vi "Outputs.vi"(8 "error in (no error)":errorcluster, 11 "State in":T1={"State"=enum."Idle", "Start Time"=timestamp(0 s since 1904-01-01), "Configuration"={"Cycle Period"=0.0, "Setpoint Entry"=0.0, "Output Device"=enum."Huber Ministat 230", "Huber Ministat 230 Settings"={"VISA resource name"="", "Simulated?"=FALSE}, "Lauda Settings"={"VISA resource name"="", "Simulated?"=FALSE, "Pump Power"=2}, "Julabo FP-50 Settings"={"VISA resource name"="", "Simulated?"=FALSE, "Pump Power"=2}, "Internal Control?"=FALSE, "Huber Unistat 410 Settings"={"VISA resource name"="", "Simulated?"=FALSE}}, "Current Time"=timestamp(0 s since 1904-01-01), "First Iteration"=FALSE, "Data"={"TCU Speed"=0.0, "Temperature"=0.0}, "Process Name"="", "TCU On?"=FALSE, "Output Error"=FALSE, "Start Log"=FALSE, "Power Level Changed"=FALSE} {"Configuration"."Julabo FP-50 Settings"."Pump Power" min=0 max=8 step=1; "Configuration"."Lauda Settings"."Pump Power" min=0 max=8 step=1}) -> (0 "error out":errorcluster, 3 "State out":T1={"State"=enum."Idle", "Start Time"=timestamp(0 s since 1904-01-01), "Configuration"={"Cycle Period"=0.0, "Setpoint Entry"=0.0, "Output Device"=enum."Huber Ministat 230", "Huber Ministat 230 Settings"={"VISA resource name"="", "Simulated?"=FALSE}, "Lauda Settings"={"VISA resource name"="", "Simulated?"=FALSE, "Pump Power"=2}, "Julabo FP-50 Settings"={"VISA resource name"="", "Simulated?"=FALSE, "Pump Power"=2}, "Internal Control?"=FALSE, "Huber Unistat 410 Settings"={"VISA resource name"="", "Simulated?"=FALSE}}, "Current Time"=timestamp(0 s since 1904-01-01), "First Iteration"=FALSE, "Data"={"TCU Speed"=0.0, "Temperature"=0.0}, "Process Name"="", "TCU On?"=FALSE, "Output Error"=FALSE, "Start Log"=FALSE, "Power Level Changed"=FALSE} {"Configuration"."Julabo FP-50 Settings"."Pump Power" min=0 max=8 step=1; "Configuration"."Lauda Settings"."Pump Power" min=0 max=8 step=1})   [LabVIEW 2018, in "TCU Module.lvlib" / "TCU Module Engine.lvlib"]
uses:
  TCU Module Engine.lvlib
  TCU State Cluster.ctl
  State Enum.ctl
  TCU Module Settings Cluster.ctl
  Output Devices.ctl
  Huber TCU/Huber Settings.ctl
  Lauda Integral XT-150 TCU/Lauda Settings.ctl
  Julabo Type 1 TCU/Julabo Type 1 TCU Folder/Julabo FP-50 Settings.ctl
  Huber Unistat 410 TCU/Huber Unistat 410 Settings.ctl
  Tag VIs/Tag FGV Operation Enum.ctl
  Shared Variables/Dynamic Shared Variables.lvlib
  Huber TCU/Huber Ministat 230 TCU.lvlib
  Lauda Integral XT-150 TCU/Lauda TCU.lvlib
  Julabo Type 1 TCU/Julabo Type 1 TCU Folder/Julabo Type FP-50 TCU.lvlib
  Huber Unistat 410 TCU/Huber Unistat 410 TCU.lvlib
  TCU Module.lvlib
panel:
  # "Output Instruments"
  # "Output Instruments"
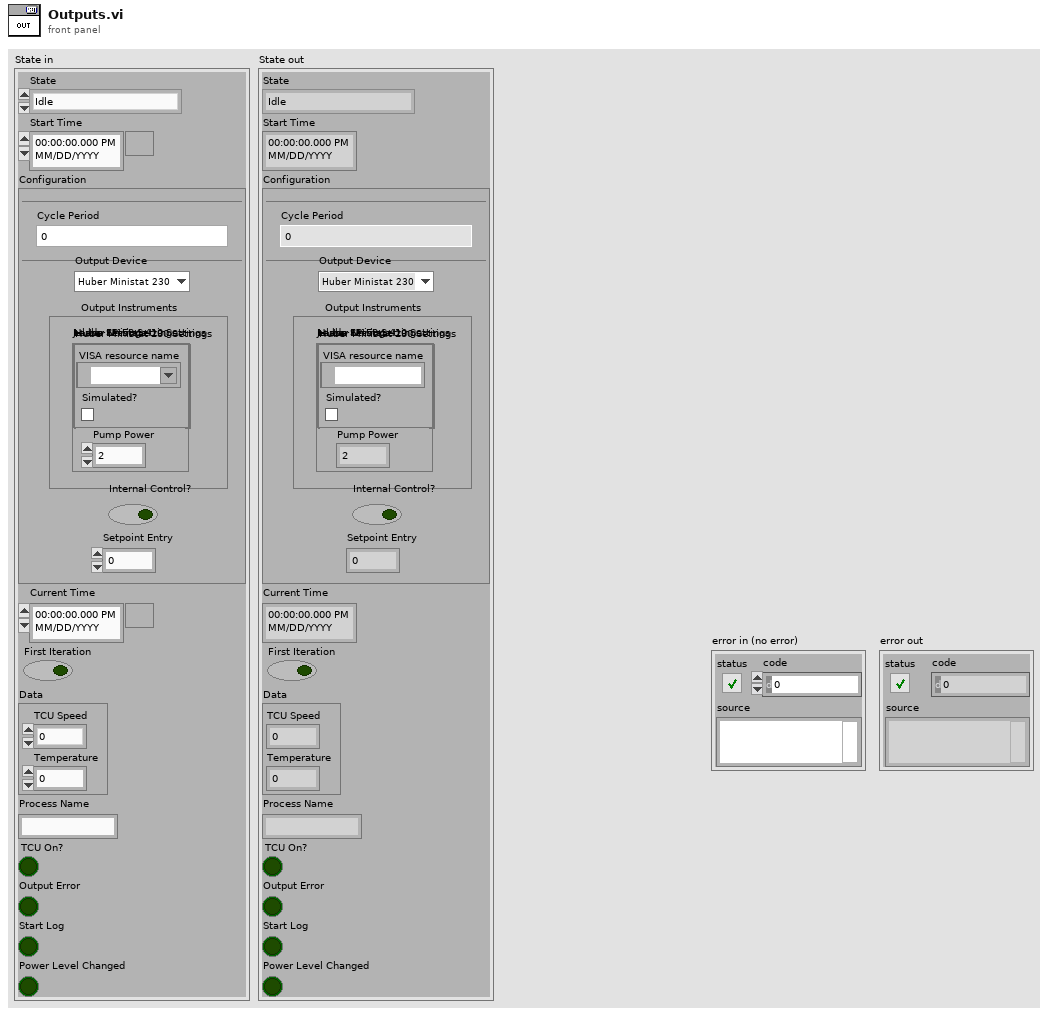
[diagram p1: front panel]
types:
  T1 = typedef "TCU Module.lvlib/TCU Module Engine.lvlib/TCU State Cluster.ctl" = cluster{"State":T2, "Start Time":timestamp, "Configuration":T3, "Current Time":timestamp, "First Iteration":bool, "Data":cluster{"TCU Speed":dbl, "Temperature":dbl}, "Process Name":string, "TCU On?":bool, "Output Error":bool, "Start Log":bool, "Power Level Changed":bool}
  T2 = typedef "TCU Module.lvlib/TCU Module Engine.lvlib/State Enum.ctl" = enum16{"Measuring", "Idle", "Paused"}
  T3 = typedef "TCU Module.lvlib/TCU Module Settings Cluster.ctl" = cluster{"Cycle Period":dbl, "Setpoint Entry":dbl, "Output Device":T4, "Huber Ministat 230 Settings":T5, "Lauda Settings":T6, "Julabo FP-50 Settings":T7, "Internal Control?":bool, "Huber Unistat 410 Settings":T8}
  T4 = typedef "Output Devices.ctl" = enum16{"Default", "Huber Ministat 230", "Huber Unistat 410", "Lauda XT-150", "Julabo FP-50"}
  T5 = typedef "Huber Ministat 230 TCU.lvlib/Huber Settings.ctl" = cluster{"VISA resource name":refnum<visa-resource-name>, "Simulated?":bool}
  T6 = typedef "Lauda TCU.lvlib/Lauda Settings.ctl" = cluster{"VISA resource name":refnum<visa-resource-name>, "Simulated?":bool, "Pump Power":i32}
  T7 = typedef "Julabo Type FP-50 TCU.lvlib/Julabo FP-50 Settings.ctl" = cluster{"VISA resource name":refnum<visa-resource-name>, "Simulated?":bool, "Pump Power":i32}
  T8 = typedef "Huber Unistat 410 TCU.lvlib/Huber Unistat 410 Settings.ctl" = cluster{"VISA resource name":refnum<visa-resource-name>, "Simulated?":bool}
  T9 = typedef "Tag FGV Operation Enum.ctl" = enum16{"Init", "Set Notification Queue", "Create Tag", "Commit", "Write Tag (Numeric)", "Write Tag (Boolean)", "Read All Tags", "Read One Tag", "Delete Tag Category", "Set Alarm Parameters (Numeric)", "Set Alarm Parameters (Boolean)", "Enable All Alarms", "Disable All Alarms", "Delete All Tags", "Read Alarms", "Ack Alarm"}
  T10 = typedef "TCU Module.lvlib/TCU Module Tag Names Cluster.ctl" = cluster{"TCU Temp":string, "Output Device Tag":string, "TCU Speed":string}
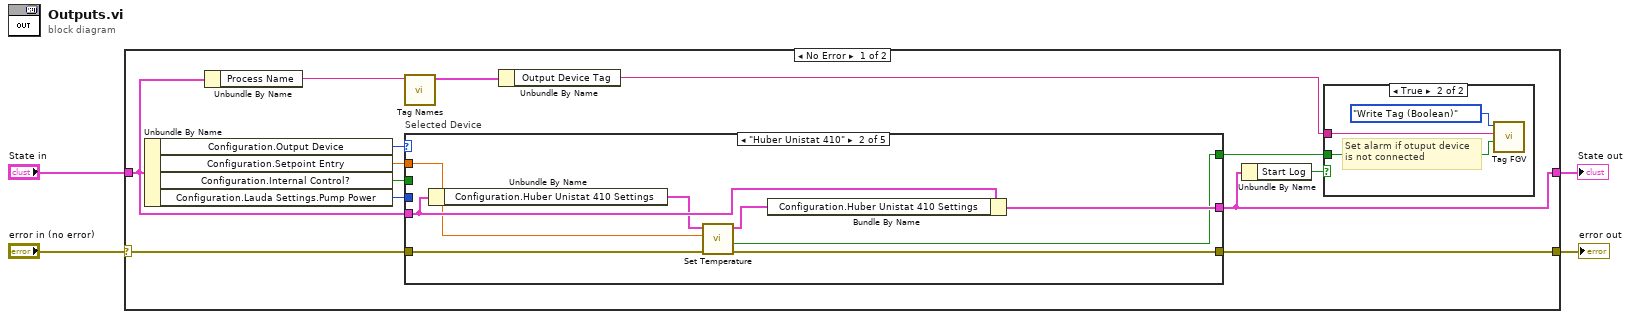
[diagram p0: block diagram]
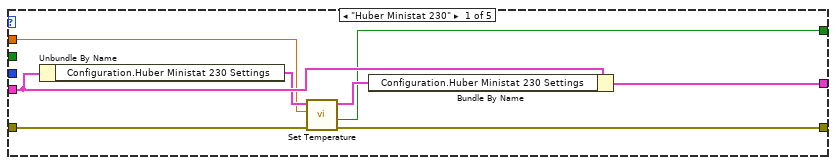
[diagram p3: hidden frame]
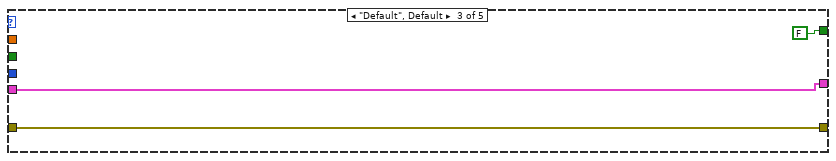
[diagram p4: hidden frame]
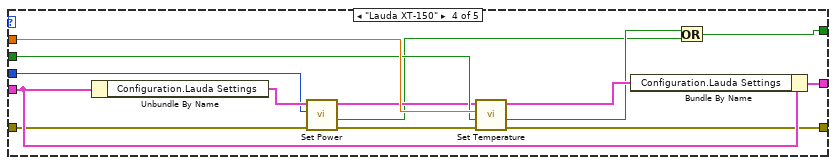
[diagram p5: hidden frame]
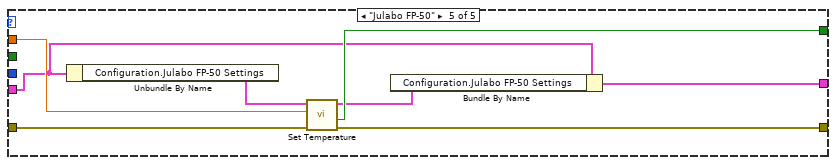
[diagram p6: hidden frame]
diagram:
  n1 = case shown="No Error" "error in (no error)" {
    selector: "error in (no error)" -> [w15 w63]
    tunnel: [w12 w63] -> w3
    tunnel: "State in" -> [w11 w62]
    tunnel: [w7 w62] -> w1
    frame No Error {
      n2 = Unbundle By Name(w11) -> ("Configuration.Output Device"=w17:T4, "Configuration.Setpoint Entry"=w16:dbl, "Configuration.Internal Control?"=w6:bool, "Configuration.Lauda Settings.Pump Power"=w5:i32)
      n3 = Unbundle By Name(w11) -> ("Process Name"=w14:string)
      n4 = call "Tag Names.vi"("Process Name"=w14) -> ("Pump Module Tag Names"=w13:T10)  [unwired: 8 in, 2 out]
      n5 = case "Selected Device" shown="\"Huber Unistat 410\"" w17 {
        tunnel: w16 -> [w21 w29 _ w51 w57]
        tunnel: w15 -> [w28 w36 w38 w45 w61]
        tunnel: [w27 w35 w38 w50 w60] -> w12
        tunnel: w11 -> [w26 w34 w39 w53 w56]
        tunnel: [w23 w31 w39 w52 w54] -> w7
        tunnel: [w22 w30 FALSE ("Connection Error") w40 w59] -> w9
        tunnel: w6 -> [_ _ _ w48 _]
        tunnel: w5 -> [_ _ _ w43 _]
        frame "Huber Ministat 230" {
          n6 = Unbundle By Name(w26) -> ("Configuration.Huber Ministat 230 Settings"=w25:T5)
          n7 = call "Set Temperature.vi"("error in (no error)"=w28, "Setpoint"=w21, "Huber Settings"=w25) -> ("error out"=w27:errorcluster, "Connection Error"=w22:bool, "Huber Settings"=w24:T5)  [unwired: 6 in]
          n8 = Bundle By Name(cluster=w26, "Configuration.Huber Ministat 230 Settings"=w24) -> (w23:T1)
        }
        frame "Huber Unistat 410" {
          n9 = Unbundle By Name(w34) -> ("Configuration.Huber Unistat 410 Settings"=w33:T8)
          n10 = call "Set Temperature.vi"("error in (no error)"=w36, "Setpoint"=w29, "Huber Settings"=w33) -> ("error out"=w35:errorcluster, "Connection Error"=w30:bool, "Huber Settings"=w32:T8)  [unwired: 6 in]
          n11 = Bundle By Name(cluster=w34, "Configuration.Huber Unistat 410 Settings"=w32) -> (w31:T1)
        }
        frame "Default", Default {
        }
        frame "Lauda XT-150" {
          n12 = Unbundle By Name(w53) -> ("Configuration.Lauda Settings"=w47:T6)
          n13 = call "Set Power.vi"("error in (no error)"=w45, "Power"=w43, "Lauda Settings"=w47) -> ("error out"=w44:errorcluster, "Connection Error"=w41:bool, "Lauda Settings"=w46:T6)  [unwired: 6 in]
          n14 = call "Set Temperature.vi"("error in (no error)"=w44, "Internal?"=w48, "Setpoint"=w51, "Lauda Settings"=w46) -> ("error out"=w50:errorcluster, "Connection Error"=w42:bool, "Lauda Settings"=w49:T6)  [unwired: 5 in]
          n15 = Bundle By Name(cluster=w53, "Configuration.Lauda Settings"=w49) -> (w52:T1)
          n16 = Or(x=w42, y=w41) -> (x .or. y?=w40:bool)
        }
        frame "Julabo FP-50" {
          n17 = Unbundle By Name(w56) -> ("Configuration.Julabo FP-50 Settings"=w58:T7)
          n18 = call "Set Temperature.vi"("error in (no error)"=w61, "Setpoint"=w57, "Julabo Fp-50 Settings"=w58) -> ("error out"=w60:errorcluster, "Connection Error"=w59:bool, "Julabo FP-50 Settings"=w55:T7)  [unwired: 6 in]
          n19 = Bundle By Name(cluster=w56, "Configuration.Julabo FP-50 Settings"=w55) -> (w54:T1)
        }
      }
      n20 = Unbundle By Name(w13) -> ("Output Device Tag"=w10:string)
      n21 = Unbundle By Name(w7) -> ("Start Log"=w8:bool)
      n22 = case shown="True" w8 {
        tunnel: w10 -> [_ w20]
        tunnel: w9 -> [_ w19]
        frame False {
        }
        frame True {
          # "Set alarm if otuput device\nis not connected"
          n23 = call "Tag FGV.vi"("Data"=w19, "Tag Name"=w20, "Operation"=Tag_FGV_Operation_Enum."Write Tag (Boolean)") -> ()  [unwired: 3 in, 6 out]
        }
      }
    }
    frame Error {
    }
  }
  "error out" <- w3
  "State out" <- w1
